vi "startSerial.vi"(8 "error in (no error)":errorcluster, 11 "TEI9150 in":refnum<class "TEI9150.lvclass">) -> (0 "error out":errorcluster, 3 "TEI9150 out":refnum<class "TEI9150.lvclass">)   [LabVIEW 2015, in "TEI9150.lvclass"]
uses:
  TEI9150.lvclass
  TEI9150.lvclass/TEI9150.ctl
  <userlib>/Common/SerialProtocols/SerialCommunicator/SerialCommunicator.lvclass
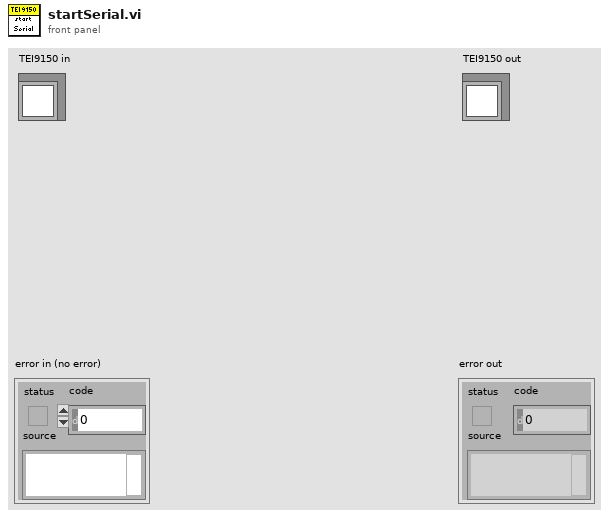
[diagram p1: front panel]
types:
  T1 = typedef "SerialProtocols.lvlib/SerialConfig.ctl" = cluster{"Serial Protocol":T2, "Protocol Parameters":T3, "Serial Message Parameters":T4}
  T2 = typedef "SerialProtocols.lvlib/SerialProtocol.ctl" = enum16{"RS232", "RS485", "SerialSimulator"}
  T3 = typedef "SerialProtocols.lvlib/ProtocolParameters.ctl" = cluster{"VISA resource name":refnum<visa-resource-name>, "Baud Rate":u32, "Data Bits":u16, "Parity":enum16{"None", "Odd", "Even", "Mark", "Space"}, "Flow Control":u16, "Stop Bits":u16, "Timeout (ms)":u32}
  T4 = typedef "SerialProtocols.lvlib/SerialMessageParameters.ctl" = cluster{"Byte Count":u32, "Enable Termination Character":bool, "Termination Char":u8}
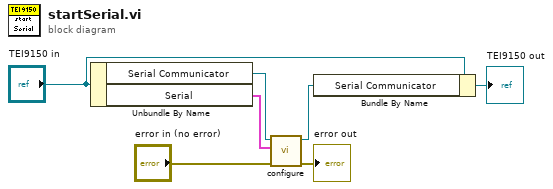
[diagram p0: block diagram]
diagram:
  n1 = Unbundle By Name("TEI9150 in") -> ("Serial Communicator"=w7:refnum<class "SerialCommunicator.lvclass">, "Serial"=w6:T1)
  n2 = call-dynamic "configure.vi"("error in (no error)"="error in (no error)", "SerialConfig"=w6, "SerialCommunicator in"=w7) -> ("error out"=→"error out":errorcluster, "SerialCommunicator out"=w3:refnum<class "SerialCommunicator.lvclass">)  [unwired: 7 in]
  n3 = Bundle By Name(cluster="TEI9150 in", "Serial Communicator"=w3) -> (→"TEI9150 out":refnum<class "TEI9150.lvclass">)
